vi "Get_Joystick_Inputs.vi"() -> (3 "All Joysticks":T1)   [LabVIEW 2012]
uses:
  Input_All_Joysticks.ctl
  Input_Single_Joystick.ctl
  <vilib>/Rock Robotics/WPI/Joystick/WPI_JoystickButtonState.ctl
  <vilib>/Rock Robotics/WPI/Joystick/WPI_JoystickGetSetRefNum.vi
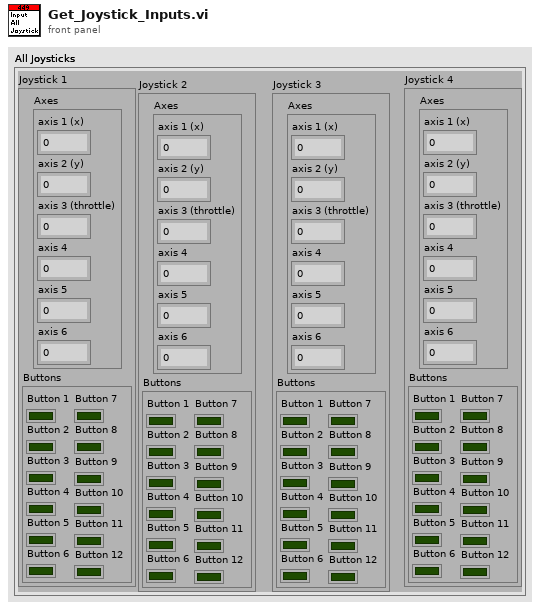
[diagram p1: front panel]
types:
  T1 = typedef "Input_All_Joysticks.ctl" = cluster{"Joystick 1":T2, "Joystick 2":T2, "Joystick 3":T2, "Joystick 4":T2}
  T2 = typedef "Input_Single_Joystick.ctl" = cluster{"Axes":cluster{"axis 1 (x)":dbl, "axis 2 (y)":dbl, "axis 3 (throttle)":dbl, "axis 4":dbl, "axis 5":dbl, "axis 6":dbl}, "Buttons":T3}
  T3 = typedef "WPI_JoystickButtonState.ctl" = cluster{"Button 1":bool, "Button 2":bool, "Button 3":bool, "Button 4":bool, "Button 5":bool, "Button 6":bool, "Button 7":bool, "Button 8":bool, "Button 9":bool, "Button 10":bool, "Button 11":bool, "Button 12":bool}
  T4 = typedef "WPI_JoystickDevRef.ctl" = cluster{"Device":T5}
  T5 = typedef "WPI_JoystickDeviceEnum.ctl" = enum16{"USB 1", "USB 2", "USB 3", "USB 4", "Kinect 1", "Kinect 2"}
  T6 = cluster{"axis 1 (x)":dbl, "axis 2 (y)":dbl, "axis 3 (throttle)":dbl, "axis 4":dbl, "axis 5":dbl, "axis 6":dbl}
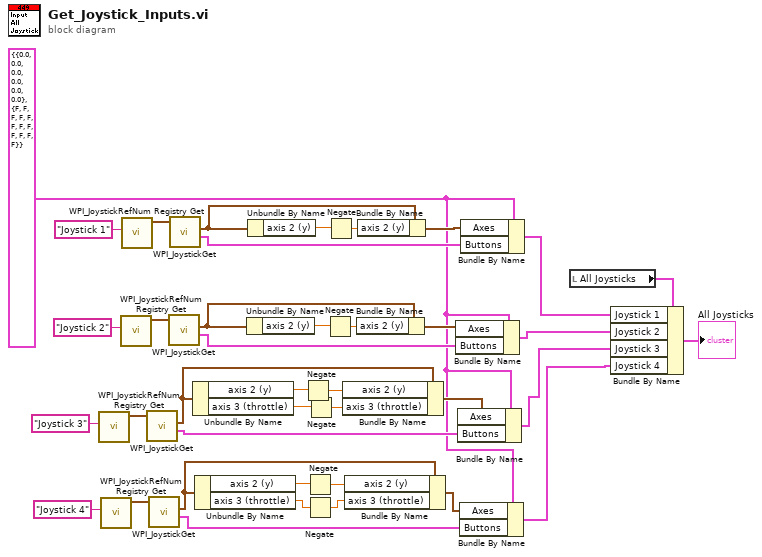
[diagram p0: block diagram]
diagram:
  w5 = T2 {"Axes"={"axis 1 (x)"=0.0, "axis 2 (y)"=0.0, "axis 3 (throttle)"=0.0, "axis 4"=0.0, "axis 5"=0.0, "axis 6"=0.0}, "Buttons"={"Button 1"=FALSE, "Button 2"=FALSE, "Button 3"=FALSE, "Button 4"=FALSE, "Button 5"=FALSE, "Button 6"=FALSE, "Button 7"=FALSE, "Button 8"=FALSE, "Button 9"=FALSE, "Button 10"=FALSE, "Button 11"=FALSE, "Button 12"=FALSE}}
  n1 = call <vilib>:"WPI_JoystickRefNum Registry Get.vi"("refnum name"="Joystick 3") -> ("JoystickDevRef"=w14:T4)  [unwired: 9 in, 1 out]
  n2 = call <vilib>:"WPI_JoystickRefNum Registry Get.vi"("refnum name"="Joystick 4") -> ("JoystickDevRef"=w15:T4)  [unwired: 9 in, 1 out]
  n3 = call <vilib>:"WPI_JoystickRefNum Registry Get.vi"("refnum name"="Joystick 2") -> ("JoystickDevRef"=w31:T4)  [unwired: 9 in, 1 out]
  n4 = call <vilib>:"WPI_JoystickRefNum Registry Get.vi"("refnum name"="Joystick 1") -> ("JoystickDevRef"=w24:T4)  [unwired: 9 in, 1 out]
  n5 = call <vilib>:"WPI_JoystickGet.vi"("JoystickDevRef"=w14) -> ("Buttons"=w19:T3, "Axes"=w13:T6)  [unwired: 4 in, 1 out]
  n6 = call <vilib>:"WPI_JoystickGet.vi"("JoystickDevRef"=w15) -> ("Buttons"=w18:T3, "Axes"=w8:T6)  [unwired: 4 in, 1 out]
  n7 = call <vilib>:"WPI_JoystickGet.vi"("JoystickDevRef"=w31) -> ("Buttons"=w37:T3, "Axes"=w28:T6)  [unwired: 4 in, 1 out]
  n8 = call <vilib>:"WPI_JoystickGet.vi"("JoystickDevRef"=w24) -> ("Buttons"=w34:T3, "Axes"=w27:T6)  [unwired: 4 in, 1 out]
  n9 = Unbundle By Name(w13) -> ("axis 2 (y)"=w21:dbl, "axis 3 (throttle)"=w1:dbl)
  n10 = Unbundle By Name(w8) -> ("axis 2 (y)"=w16:dbl, "axis 3 (throttle)"=w3:dbl)
  n11 = Unbundle By Name(w28) -> ("axis 2 (y)"=w30:dbl)
  n12 = Unbundle By Name(w27) -> ("axis 2 (y)"=w25:dbl)
  n13 = Negate(x=w21) -> (-x=w12:dbl)
  n14 = Negate(x=w16) -> (-x=w11:dbl)
  n15 = Negate(x=w3) -> (-x=w4:dbl)
  n16 = Negate(x=w1) -> (-x=w2:dbl)
  n17 = Negate(x=w30) -> (-x=w29:dbl)
  n18 = Negate(x=w25) -> (-x=w26:dbl)
  n19 = Bundle By Name(cluster=w13, "axis 2 (y)"=w12, "axis 3 (throttle)"=w2) -> (w10:T6)
  n20 = Bundle By Name(cluster=w8, "axis 2 (y)"=w11, "axis 3 (throttle)"=w4) -> (w9:T6)
  n21 = Bundle By Name(cluster=w28, "axis 2 (y)"=w29) -> (w36:T6)
  n22 = Bundle By Name(cluster=w27, "axis 2 (y)"=w26) -> (w33:T6)
  n23 = Bundle By Name(cluster=w5, "Axes"=w36, "Buttons"=w37) -> (w38:T2)
  n24 = Bundle By Name(cluster=w5, "Axes"=w10, "Buttons"=w19) -> (w7:T2)
  n25 = Bundle By Name(cluster=w5, "Axes"=w9, "Buttons"=w18) -> (w6:T2)
  n26 = Bundle By Name(cluster=w5, "Axes"=w33, "Buttons"=w34) -> (w35:T2)
  n27 = local read "All Joysticks"() -> (w22:T1)
  n28 = Bundle By Name(cluster=w22, "Joystick 1"=w35, "Joystick 2"=w38, "Joystick 3"=w7, "Joystick 4"=w6) -> (→"All Joysticks":T1)
